vi "Get Trace (example).vi"() -> ()   [LabVIEW 2016, in "LV-Data.PGSQL.lvclass"]
uses:
  LV-Data.PGSQL.lvclass
panel:
  in  "time interval":T1
  in  "max points":i32
  out "XY Graph":cluster{timestamp[], dbl[]}(graph)
  in  "path table:column":string
  out "Data.PG":refnum<class "LV-Data.PGSQL.lvclass">
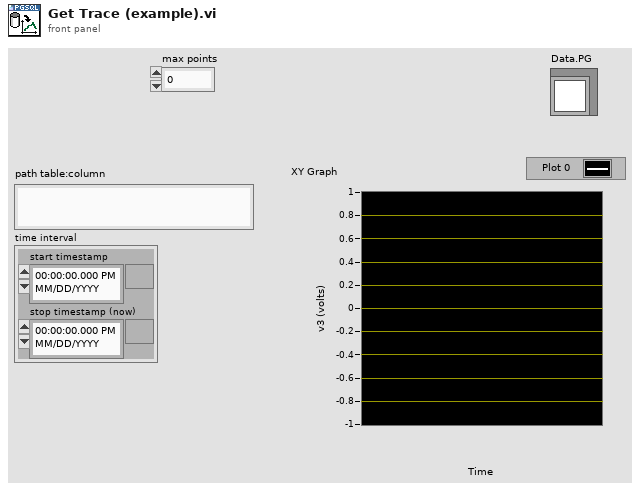
[diagram p1: front panel]
types:
  T1 = cluster{"start timestamp":timestamp, "stop timestamp (now)":timestamp}
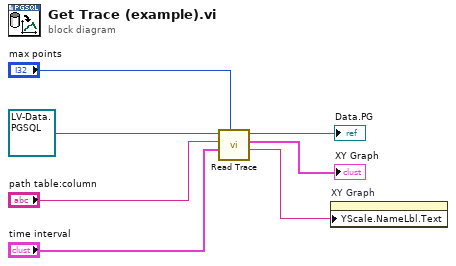
[diagram p0: block diagram]
diagram:
  n1 = call "Read Trace.vi"("max points (-1 = all)"="max points", "time interval"="time interval", "PG path"="path table:column", "Data.PGQL in"=refnum<class "LV-Data.PGSQL.lvclass"> refnum ("Data.PG in")) -> ("Column (units)"=w6:string, "Trace"=→"XY Graph":cluster{timestamp[], dbl[]}, "Data.PGSQL out"=→"Data.PG":refnum<class "LV-Data.PGSQL.lvclass">)  [unwired: 3 in, 2 out]
  n2 = property on="XY Graph" class="XYGraph (strict)"("YScale.NameLbl.Text"=w6) -> ()  [unwired: 2 in, 2 out]
